vi "FeedBack Chanel.vi"(0 "Test Name":string, 5 "Channels (Int)":i32[](array[numeric]), 7 "FeedBack Channel":string[](array[string])=["fgdgfvcbc", "vnfhgjkn", "21354682"], 9 "Wait/Poll (ms)":u32, 11 "Parameter":u8) -> (4 "Out":i32, 6 "Array":bool[](array[boolean]), 10 "Fail":bool, 12 "Input Status":bool[](array[boolean]), 13 "Channel No":i32[](array[numeric]))   [LabVIEW 2015]
uses:
  Galobal variable_TI.vi
  Project Setup/Globle Variable/GR_Servo.vi
panel:
  out "Pokayoka Result":cluster{"Sensor Name":string, "Boolean":bool}[](array[cluster])
  out "output array":bool[](array[boolean])
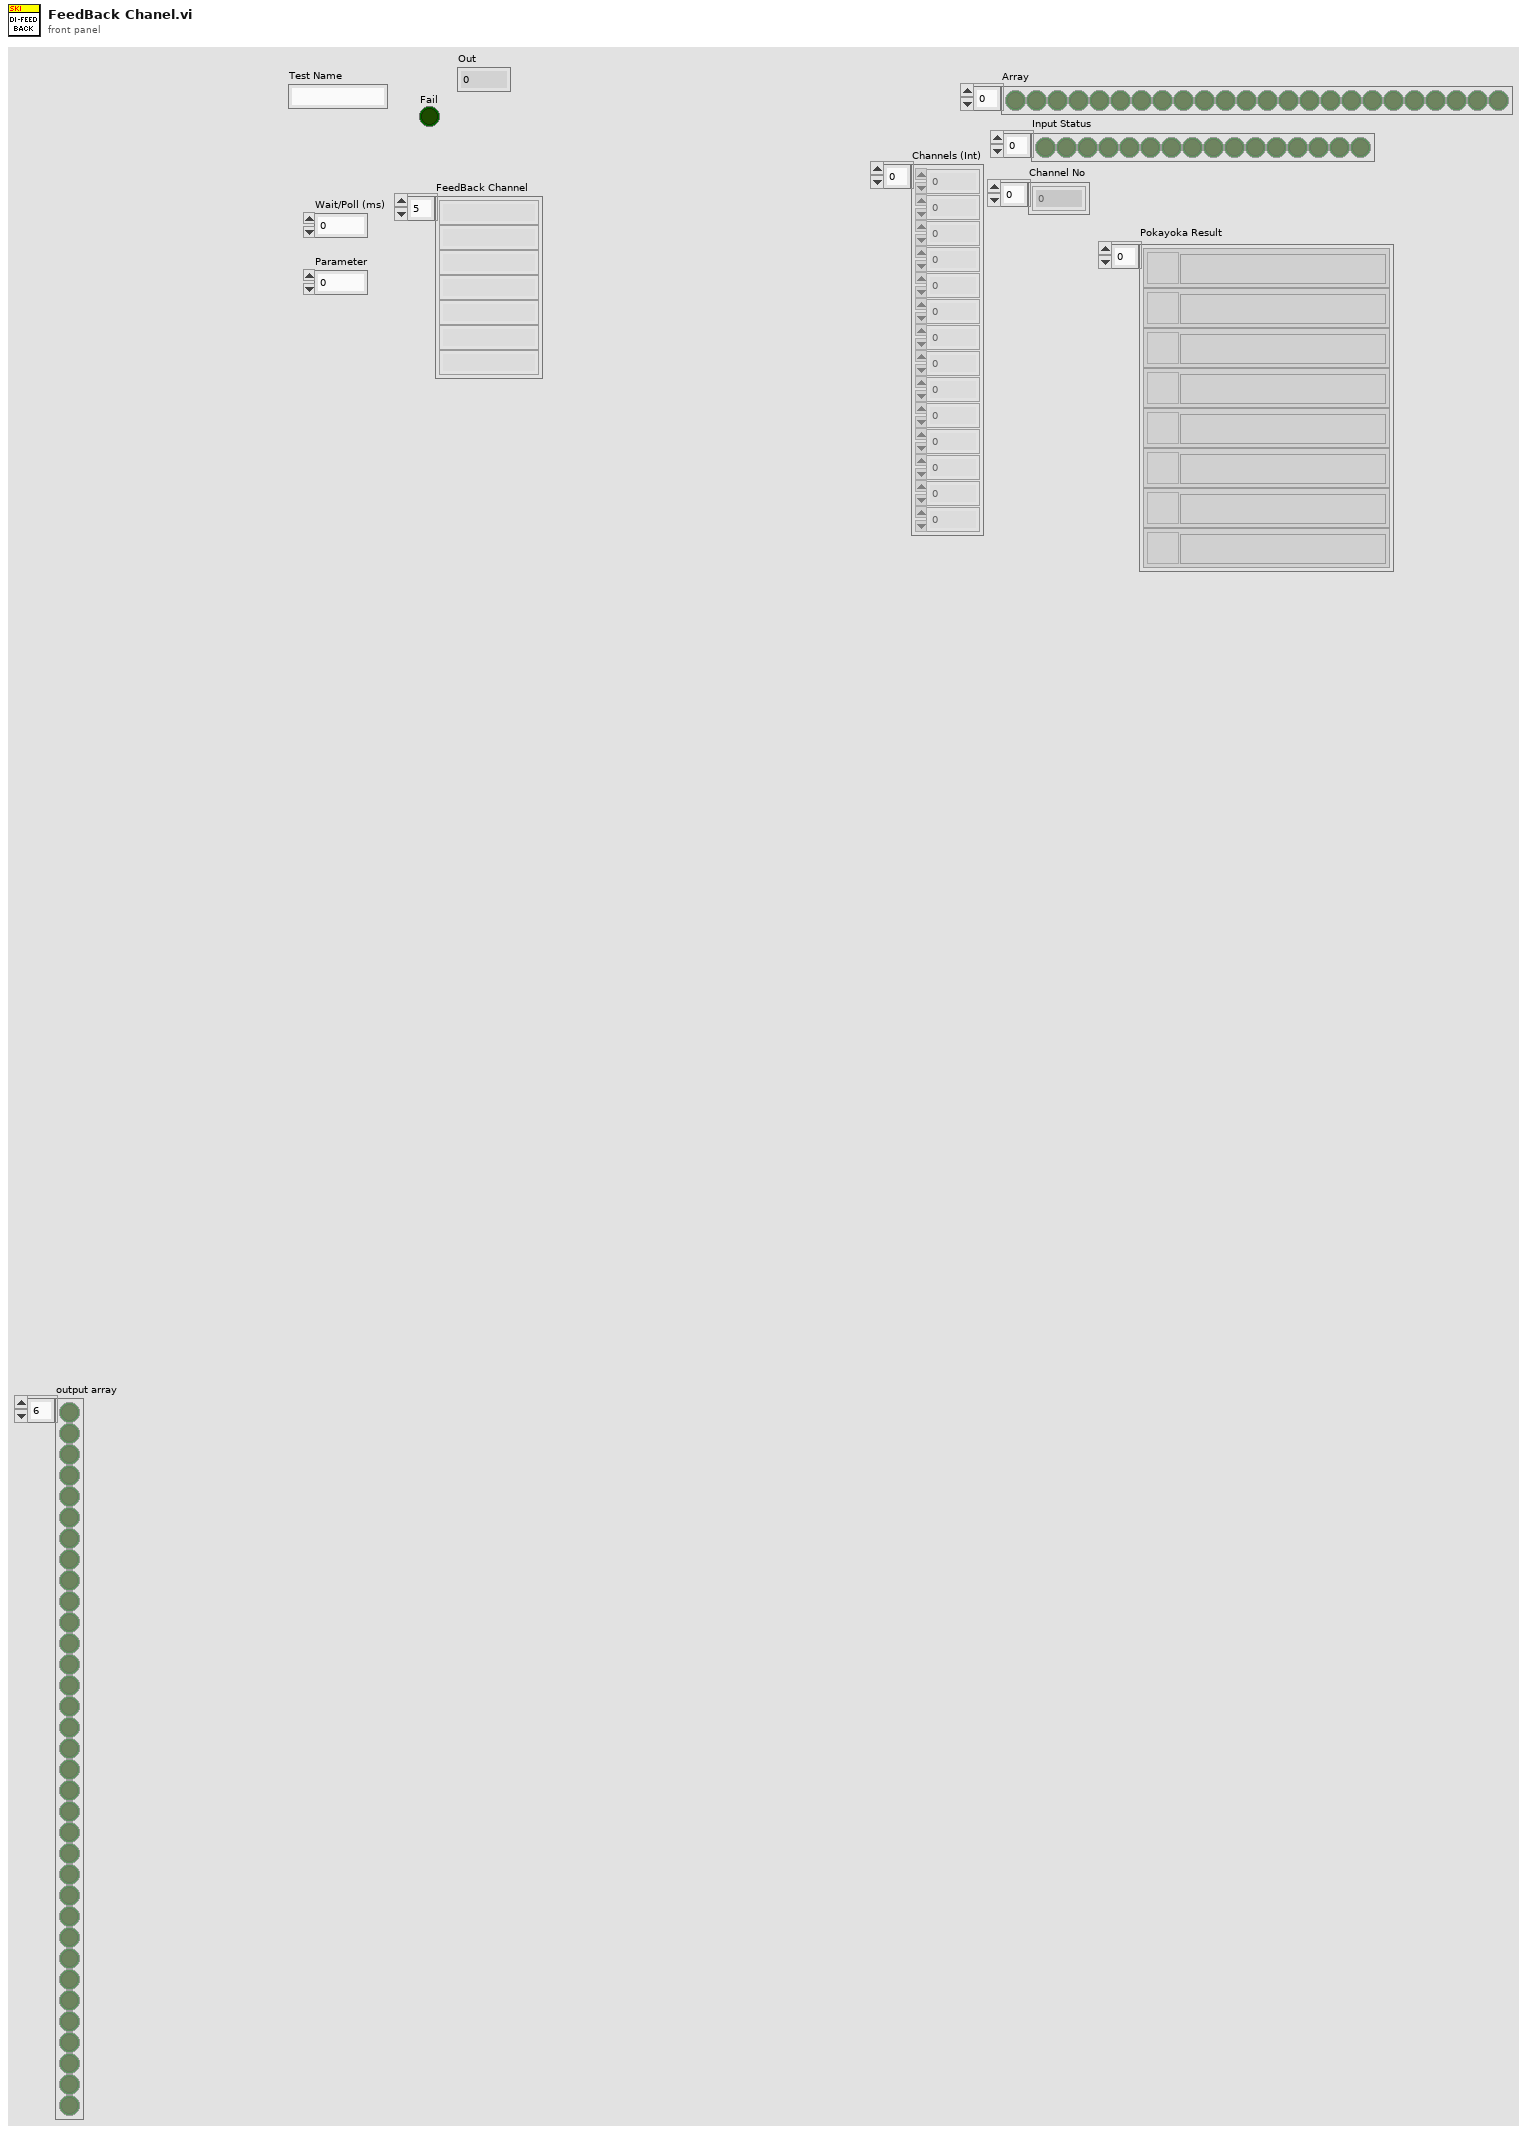
[diagram p1: front panel]
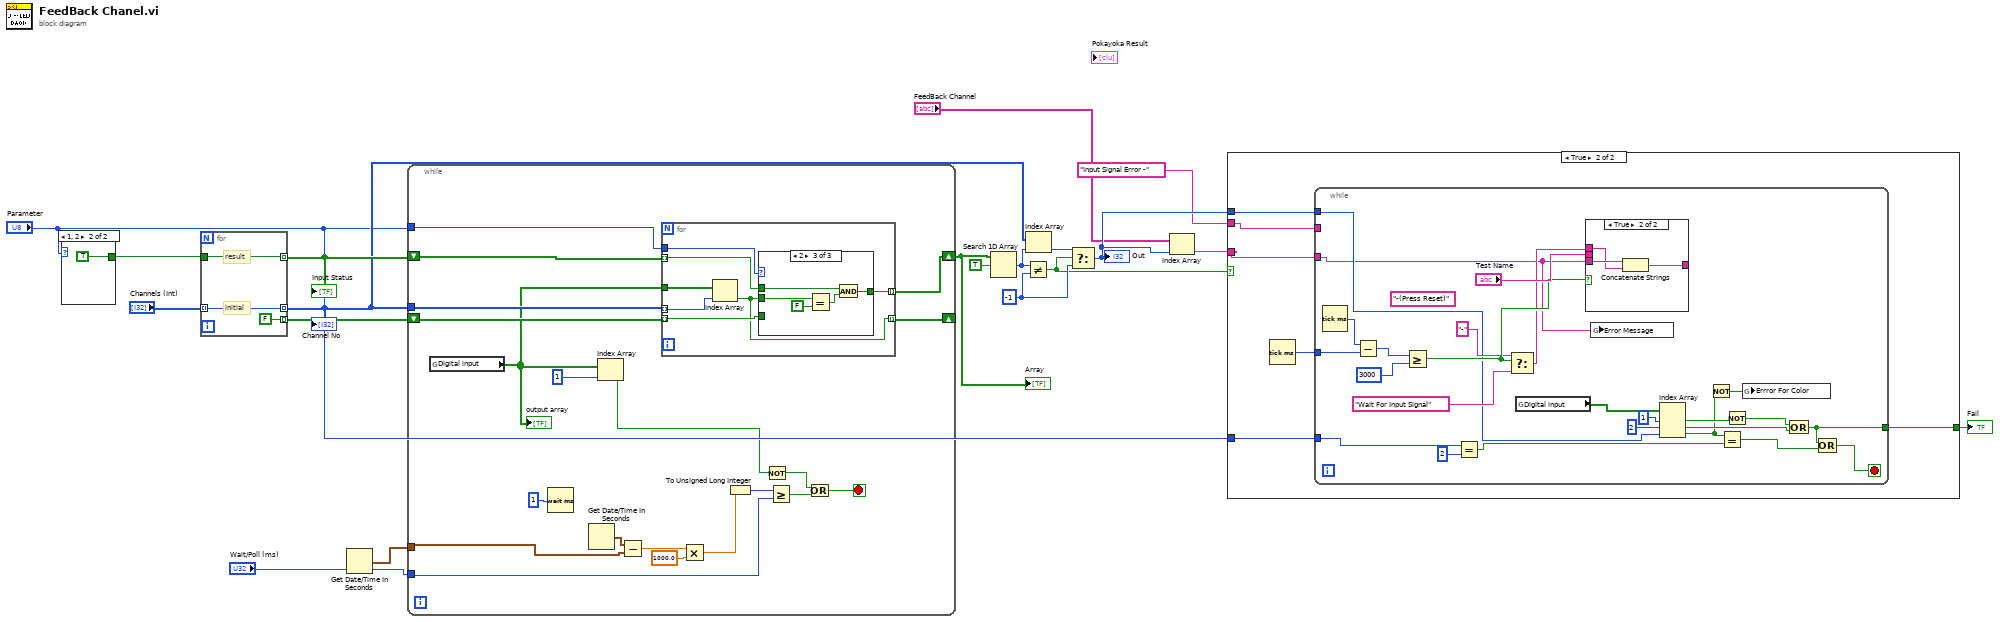
[diagram p0: block diagram]
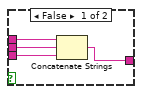
[diagram p3: hidden frame]
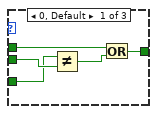
[diagram p4: hidden frame]
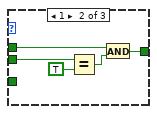
[diagram p5: hidden frame]
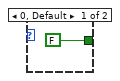
[diagram p6: hidden frame]
diagram:
  w19 = -1 ("y")
  n1 = case shown="1, 2" "Parameter" {
    tunnel: [FALSE TRUE] -> w10
    frame 0, Default {
    }
    frame 1, 2 {
    }
  }
  n2 = for {
    tunnel: [w24] -> w5 mode=indexing
    tunnel: w10 -> [w24]
    tunnel: "Channels (Int)" -> [w23] mode=indexing
    tunnel: [w23] -> w4 mode=indexing
    tunnel: [FALSE] -> w14 mode=indexing
    # "result"
    # "initial"
  }
  "Input Status" <- w5
  "Channel No" <- w4
  n3 = Get Date/Time In Seconds() -> (seconds since 1Jan1904=w13:timestamp)
  n4 = while {
    tunnel: "Wait/Poll (ms)" -> [w29]
    tunnel: w13 -> [w43]
    tunnel: w4 -> [w38]
    tunnel: "Parameter" -> [w37]
    shift-right: [w36] -> w16
    shift-left: w5 -> [w34]
    shift-right: [w35] -> _
    shift-left: w14 -> [w33]
    stop <- w31 stop-if-true
    n5 = global read "Galobal variable_TI.vi" "Digital input"() -> (w25:bool[])
    "output array" <- w25
    n6 = Wait (ms)(milliseconds to wait=u32 1) -> ()  [unwired: 1 out]
    n7 = Get Date/Time In Seconds() -> (seconds since 1Jan1904=w44:timestamp)
    n8 = Index Array(array=w25, index=1) -> (element=w27:bool)
    n9 = Subtract(x=w44, y=w43) -> (x-y=w42:dbl)
    n10 = for {
      tunnel: w33 -> [w46] mode=indexing
      tunnel: w34 -> [w48] mode=indexing
      tunnel: w25 -> [w51]
      tunnel: w38 -> [w50] mode=indexing
      tunnel: w37 -> [w49]
      tunnel: [w47] -> w36 mode=indexing
      tunnel: [w45] -> w35 mode=indexing
      n11 = Index Array(array=w51, index=w50) -> (element=w45:bool)
      n12 = case shown="2" w49 {
        tunnel: w45 -> [w56 w59 w66]
        tunnel: w48 -> [w54 w58 w63]
        tunnel: [w52 w57 w62] -> w47
        tunnel: w46 -> [w55 _ _]
        frame 0, Default {
          n13 = Not Equal?(x=w55, y=w56) -> (x != y?=w53:bool)
          n14 = Or(x=w54, y=w53) -> (x .or. y?=w52:bool)
        }
        frame 1 {
          n15 = Equal?(x=w59, y=TRUE) -> (x = y?=w60:bool)
          n16 = And(x=w58, y=w60) -> (x .and. y?=w57:bool)
        }
        frame 2 {
          n17 = Equal?(x=w66, y=FALSE) -> (x = y?=w64:bool)
          n18 = And(x=w63, y=w64) -> (x .and. y?=w62:bool)
        }
      }
    }
    n19 = Multiply(x=w42, y=1000.0) -> (x*y=w40:dbl)
    n20 = To Unsigned Long Integer(number=w40) -> (unsigned 32bit integer=w39:u32)
    n21 = Not(x=w27) -> (.not. x?=w28:bool)
    n22 = Greater Or Equal?(x=w39, y=w29) -> (x >= y?=w32:bool)
    n23 = Or(x=w28, y=w32) -> (x .or. y?=w31:bool)
  }
  "Array" <- w16
  n24 = Search 1D Array(1D array=w16, element=TRUE) -> (index of element=w17:i32)  [unwired: 1 in]
  n25 = Not Equal?(x=w17, y=w19) -> (x != y?=w9:bool)
  n26 = Index Array(array=w4, index=w17) -> (element=w18:i32)
  n27 = Select(t=w18, s=w9, f=w19) -> (s? t:f=w8:i32)
  "Out" <- w8
  n28 = Index Array(array="FeedBack Channel", index=w8) -> (element=w7:string)
  n29 = case shown="True" w9 {
    tunnel: w8 -> [_ w69]
    tunnel: w7 -> [_ w72]
    tunnel: "Input Signal Error -" ("string") -> [_ w71]
    tunnel: "Parameter" -> [_ w68]
    tunnel: [_ w67] -> w1
    frame False {
    }
    frame True {
      n30 = Tick Count (ms)() -> (millisecond timer value=w70:u32)
      n31 = while {
        tunnel: w72 -> [w75]
        tunnel: w71 -> [_]
        tunnel: w70 -> [w95]
        tunnel: w69 -> [w81]
        tunnel: w68 -> [w80]
        tunnel: [w78] -> w67
        stop <- w82 stop-if-true
        (unwired) "-(Press Reset)" ("f")
        n32 = Tick Count (ms)() -> (millisecond timer value=w96:u32)
        n33 = Subtract(x=w96, y=w95) -> (x-y=w94:u32)
        n34 = Greater Or Equal?(x=w94, y=u32 3000) -> (x >= y?=w92:bool)
        n35 = Equal?(x=w80, y=u8 2) -> (x = y?=w77:bool)
        n36 = Select(t="-" ("f"), s=w92, f="Wait For Input Signal") -> (s? t:f=w91:string)
        n37 = global read "Galobal variable_TI.vi" "Digital input"() -> (w87:bool[])
        n38 = case shown="True" w92 {
          tunnel: w75 -> [w101 w104]
          tunnel: "Test Name" -> [w100 _]
          tunnel: w91 -> [w99 w103]
          tunnel: [w98 w102] -> _
          frame False {
            n39 = Concatenate Strings(w99, w100, w101) -> (w98:string)
          }
          frame True {
            n40 = Concatenate Strings(w104, w103) -> (w102:string)
          }
        }
        n41 = global write "GR_Servo.vi" "Error Message"(w75) -> ()
        n42 = Index Array(array=w87, index #1=1 ("index"), index #2=2 ("index"), index #3=w81) -> (element #1=w86:bool, element #2=w83:bool, element #3=w74:bool)
        n43 = Not(x=w74) -> (.not. x?=w73:bool)
        n44 = Equal?(x=w74, y=w77) -> (x = y?=w76:bool)
        n45 = Not(x=w86) -> (.not. x?=w84:bool)
        n46 = global write "Galobal variable_TI.vi" "Errror For Color"(w73) -> ()
        n47 = Compound Arithmetic op=OR(w84, w83) -> (w78:bool)
        n48 = Compound Arithmetic op=OR(w78, w76) -> (w82:bool)
      }
    }
  }
  "Fail" <- w1
